vi "Do Bake.vi"(8 "error in (no error)":errorcluster, 11 "Chef in":refnum<class "Chef.lvclass">) -> (0 "error out":errorcluster, 3 "Chef out":refnum<class "Chef.lvclass">)   [LabVIEW 2011, in "Chef.lvclass"]
uses:
  Chef.lvclass
  Chef.lvclass/Chef.ctl
  Appliance/Appliance.lvclass
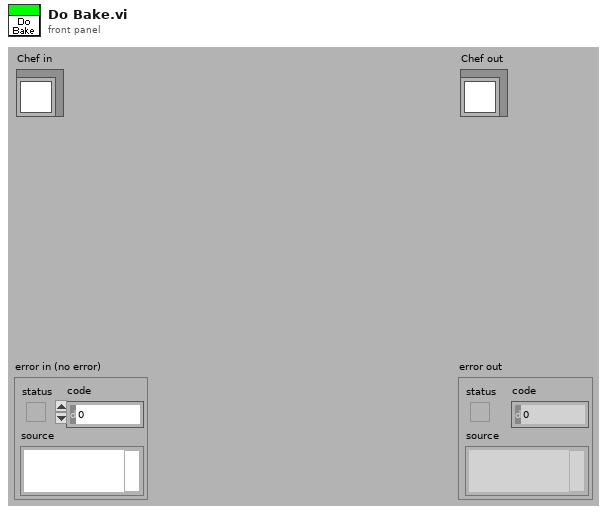
[diagram p1: front panel]
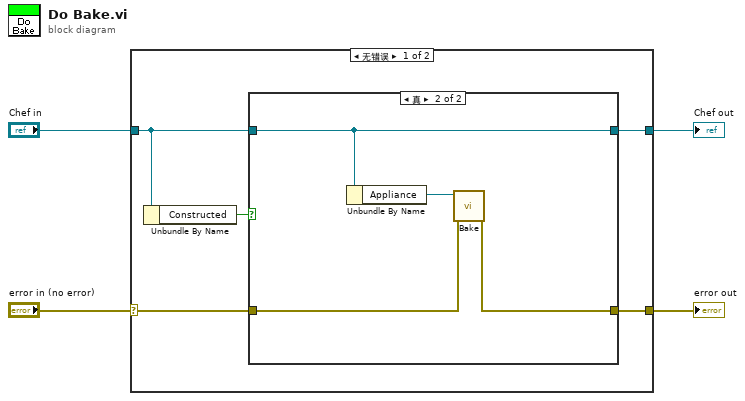
[diagram p0: block diagram]
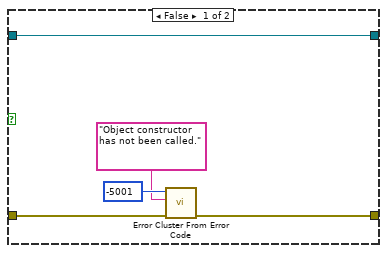
[diagram p2: hidden frame]
diagram:
  n1 = case shown="无错误" "error in (no error)" {
    selector: "error in (no error)" -> [w9 w20]
    tunnel: [w8 w20] -> w3
    tunnel: [w7 w19] -> w1
    tunnel: "Chef in" -> [w6 w19]
    frame No Error {
      n2 = Unbundle By Name(w6) -> ("Constructed"=w5:bool)
      n3 = case shown="真" w5 {
        tunnel: w6 -> [w13 w15]
        tunnel: w9 -> [w14 w17]
        tunnel: [w12 w16] -> w8
        tunnel: [w13 w15] -> w7
        frame False {
          n4 = call <vilib>:"Error Cluster From Error Code.vi"("error in (no error)"=w14, "error message (\"\")"="Object constructor has not been called." ("error message (\"\")"), "error code (0)"=-5001) -> ("error out"=w12:errorcluster)  [unwired: 6 in]
        }
        frame True {
          n5 = Unbundle By Name(w15) -> ("Appliance"=w18:refnum<class "Appliance.lvclass">)
          n6 = call-dynamic "Bake.vi"("error in (no error)"=w17, "Appliance in"=w18) -> ("error out"=w16:errorcluster)  [unwired: 8 in, 1 out]
        }
      }
    }
    frame Error {
    }
  }
  "error out" <- w3
  "Chef out" <- w1
